vi "Get_Next_Data.vi"(8 "error in (no error)":errorcluster caption="entrée d'erreur (pas d'erreur)", 11 "Firebase Benches en entrée":refnum<class "Firebase Scan.lvclass">) -> (0 "error out":errorcluster caption="sortie d'erreur", 3 "Firebase Benches en sortie":refnum<class "Firebase Scan.lvclass">)   [LabVIEW 2020, in "Library Instrument & Equipement.lvlib" / "Library FireBase.lvlib" / "Firebase Scan.lvclass"]
doc: "Returns data according to Value_To_Find Use Nb_To_Read to determine the number to read\nPlease initialise the following values before use the VI\n - Name BDD\n - Value to find\n - Document\n - API Key"
uses:
  Firebase Scan.lvclass
  C:/Users/ngarcin/OneDrive - Altyor/Standard TB/Class/Firebase/Source/Firebase Driver/Firebase Driver.lvclass
  Firebase Scan.lvclass/Firebase Scan.ctl
  JSON API/JSON Value/Set from JSON string.vi
  JSON API/JSON Value/JSON Value.lvclass
  Firebase Altyor/Firebase Altyor.lvclass
  JSON API/Variant JSON/Variant JSON.lvlib
  JSON API/Get Polymorphic/JSON GetSet.lvlib
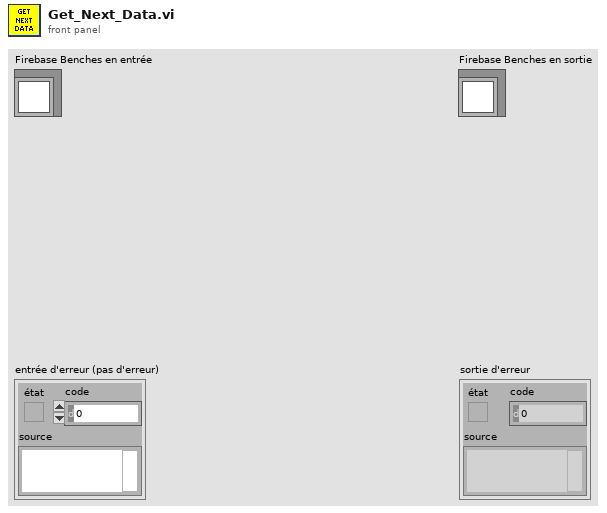
[diagram p1: front panel]
types:
  T1 = cluster{"name":string, "fields":cluster{"Result":cluster{"booleanValue":bool}, "CreationDate":cluster{"timestampValue":string}, "Batch":cluster{"stringValue":string}, "SerialNumber":cluster{"stringValue":string}, "EndOfProduction":cluster{"timestampValue":string}, "FW_Version":cluster{"mapValue":cluster{"fields":cluster{"Bootloader":cluster{"mapValue":cluster{"fields":cluster{"File_Name":cluster{"stringValue":string}, "Version":cluster{"mapValue":cluster{"fields":cluster{"Major":cluster{"stringValue":string}, "Minor":cluster{"stringValue":string}}}}, "Checksum":cluster{"stringValue":string}}}}, "SoftDevice":cluster{"mapValue":cluster{"fields":cluster{"File_Name":cluster{"stringValue":string}, "Version":cluster{"mapValue":cluster{"fields":cluster{"Major":cluster{"stringValue":string}, "Minor":cluster{"stringValue":string}}}}, "Checksum":cluster{"stringValue":string}}}}, "DFU":cluster{"mapValue":cluster{"fields":cluster{"File_Name":cluster{"stringValue":string}, "Version":cluster{"mapValue":cluster{"fields":cluster{"Major":cluster{"stringValue":string}, "Minor":cluster{"stringValue":string}}}}, "Checksum":cluster{"stringValue":string}}}}}}}, "PartNumber":cluster{"stringValue":string}, "OrderNumber":cluster{"stringValue":string}, "Operator":cluster{"stringValue":string}, "Deleted":cluster{"booleanValue":bool}}}[]
  T2 = cluster{"documents":cluster{"name":string, "fields":cluster{"Result":cluster{"booleanValue":bool}, "CreationDate":cluster{"timestampValue":string}, "Batch":cluster{"stringValue":string}, "SerialNumber":cluster{"stringValue":string}, "EndOfProduction":cluster{"timestampValue":string}, "FW_Version":cluster{"mapValue":cluster{"fields":cluster{"Bootloader":cluster{"mapValue":cluster{"fields":cluster{"File_Name":cluster{"stringValue":string}, "Version":cluster{"mapValue":cluster{"fields":cluster{"Major":cluster{"stringValue":string}, "Minor":cluster{"stringValue":string}}}}, "Checksum":cluster{"stringValue":string}}}}, "SoftDevice":cluster{"mapValue":cluster{"fields":cluster{"File_Name":cluster{"stringValue":string}, "Version":cluster{"mapValue":cluster{"fields":cluster{"Major":cluster{"stringValue":string}, "Minor":cluster{"stringValue":string}}}}, "Checksum":cluster{"stringValue":string}}}}, "DFU":cluster{"mapValue":cluster{"fields":cluster{"File_Name":cluster{"stringValue":string}, "Version":cluster{"mapValue":cluster{"fields":cluster{"Major":cluster{"stringValue":string}, "Minor":cluster{"stringValue":string}}}}, "Checksum":cluster{"stringValue":string}}}}}}}, "PartNumber":cluster{"stringValue":string}, "OrderNumber":cluster{"stringValue":string}, "Operator":cluster{"stringValue":string}, "Deleted":cluster{"booleanValue":bool}}}[], "nextPageToken":string}
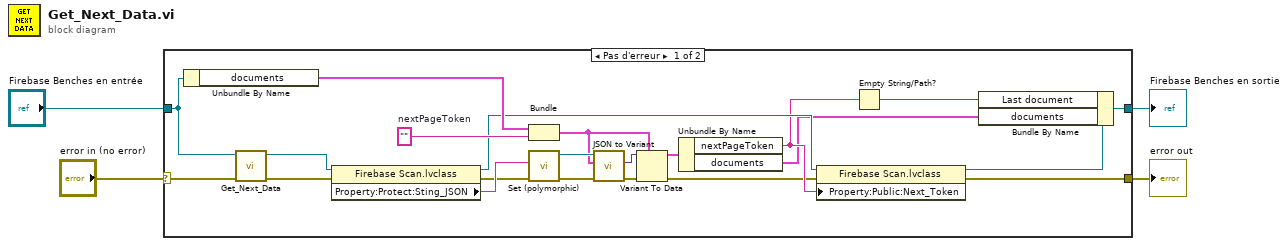
[diagram p0: block diagram]
diagram:
  n1 = case shown="Pas d'erreur" "error in (no error)" {
    selector: "error in (no error)" -> [w9 w27]
    tunnel: "Firebase Benches en entrée" -> [w6 w28]
    tunnel: [w10 w28] -> w3
    tunnel: [w13 w27] -> w2
    frame No Error {
      w21 = ""  # nextPageToken
      n2 = Unbundle By Name(w6) -> ("documents"=w20:T1)
      n3 = call-parent "Get_Next_Data.vi"("error in (no error)"=w9, "Firebase Altyor en entrée"=w6) -> ("error out"=w8:errorcluster, "Firebase Altyor en sortie"=w7:refnum<class "Firebase Scan.lvclass">)  [unwired: 8 in]
      n4 = property class="Firebase Scan.lvclass"(reference=w7, error in=w8) -> (reference out=w18:refnum<class "Firebase Scan.lvclass">, error out=w12:errorcluster, "Property:Protect:Sting_JSON"=w23:string)
      n5 = Bundle("documents"=w20, "nextPageToken"=w21) -> (w19:T2)  [unwired: 1 in]
      n6 = call-poly "Set (polymorphic).vi"("error in (no error)"=w12, "JSON stream"=w23) -> ("error out"=w24:errorcluster, "JSON Value out"=w26:refnum<class "JSON Value.lvclass">)  [unwired: 7 in, 1 out]
      n7 = call "JSON to Variant.vi"("error in (no error)"=w24, "Variant (Data Type)"=w19, "JSON Value"=w26) -> ("error out"=w25:errorcluster, "Variant out"=w5:variant)  [unwired: 7 in]
      n8 = Variant To Data(error in=w25, type=w19, Variant=w5) -> (data=w22:T2, error out=w11:errorcluster)
      n9 = Unbundle By Name(w22) -> ("nextPageToken"=w17:string, "documents"=w15:T1)
      n10 = property class="Firebase Scan.lvclass"(reference=w18, error in=w11, "Property:Public:Next_Token"=w17) -> (reference out=w16:refnum<class "Firebase Scan.lvclass">, error out=w13:errorcluster)
      n11 = Empty String/Path?(string/path=w17) -> (empty?=w14:bool)
      n12 = Bundle By Name(cluster=w16, "Last document"=w14, "documents"=w15) -> (w10:refnum<class "Firebase Scan.lvclass">)
    }
    frame Error {
    }
  }
  "Firebase Benches en sortie" <- w3
  "error out" <- w2
